vi "Write File.vi"(7 "File ID":string, 8 "error in (no error)":errorcluster, 9 "Segment 1 to 99":T3(array[cluster]), 10 "Segment 0":T2={"Start"=enum."Upward PV tart", "Cycle data"=999, "Pattern link data"=0, "Tag data"="PROG551A"}, 11 "Serial Config":T1={"串口选择"="", "通讯速率"=9600, "超时时间"=200, "数据位长"=8, "奇偶校验"=enum."None", "停止位长"=10, "握手控制"=0, "字符结束"=TRUE, "结束字符"=10, "仪器地址"=1} {"结束字符" format="%.0x"; "握手控制" items=["None", "XON/XOFF", "RTS/CTS", "XON/XOFF & RTS/CTS", "DTR/DSR", "XON/XOFF & DTR/DSR"]; "停止位长" items=["1.0"=10, "1.5"=15, "2.0"=20]; "数据位长" min=5 max=8 step=1}) -> (0 "error out":errorcluster)   [LabVIEW 2010, in "DCP551.lvlib"]
uses:
  DCP551.lvlib
  <vilib>/Instr/_visa.llb/VISA Configure Serial Port (Instr).vi
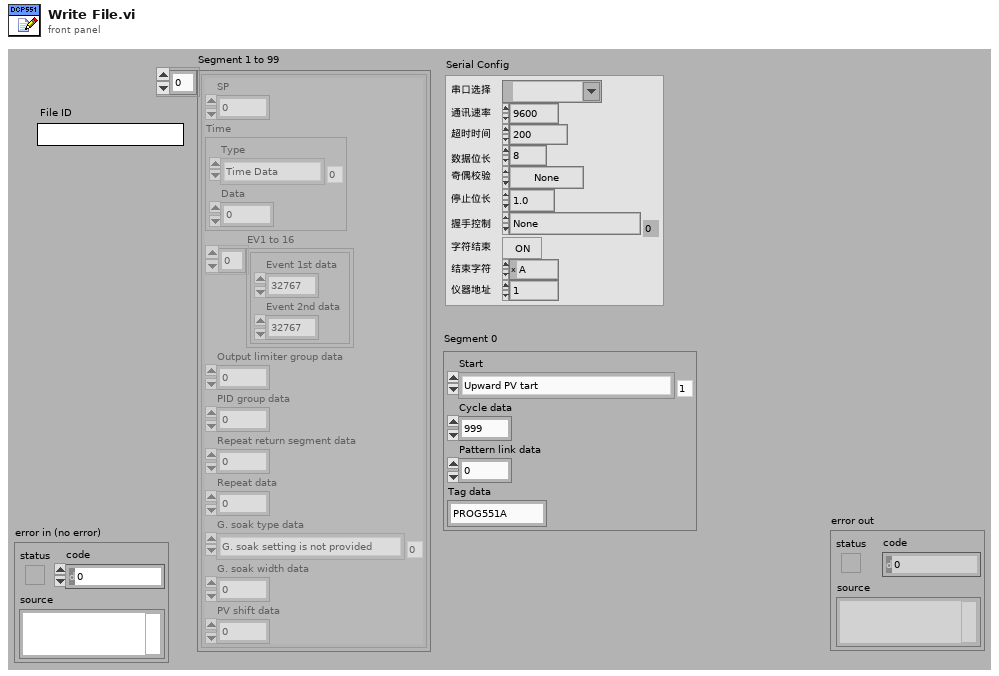
[diagram p1: front panel]
types:
  T1 = cluster{"串口选择":refnum<visa-resource-name>, "通讯速率":u32, "超时时间":u32, "数据位长":u16, "奇偶校验":enum16{"None", "Odd", "Even", "Mark", "Space"}, "停止位长":u16, "握手控制":u16, "字符结束":bool, "结束字符":u8, "仪器地址":u32}
  T2 = cluster{"Start":enum16{"Non PV start", "Upward PV tart", "Downward PV start", "Either upward of downward PV start"}, "Cycle data":i32, "Pattern link data":i32, "Tag data":string}
  T3 = cluster{"SP":dbl, "Time":cluster{"Type":enum16{"Time Data", "delta Dtada", "SP Data"}, "Data":i32}, "EV1 to 16":cluster{"Event 1st data":i32, "Event 2nd data":i32}[], "Output limiter group data":i32, "PID group data":i32, "Repeat return segment data":i32, "Repeat data":i32, "G. soak type data":enum16{"G. soak setting is not provided", "Segment start point", "Segment end point", "Total segment"}, "G. soak width data":i32, "PV shift data":i32}[]
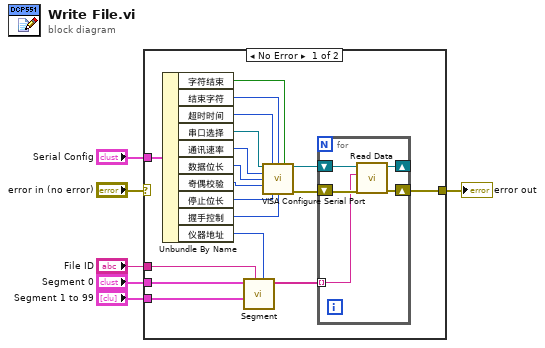
[diagram p0: block diagram]
diagram:
  n1 = case shown="No Error" "error in (no error)" {
    selector: "error in (no error)" -> [_ w30]
    tunnel: "Serial Config" -> [w15 _]
    tunnel: [w12 w30] -> w5
    tunnel: "Segment 1 to 99" -> [w10 _]
    tunnel: "Segment 0" -> [w11 _]
    tunnel: "File ID" -> [w9 _]
    frame No Error {
      n2 = Unbundle By Name(w15) -> ("字符结束"=w18:bool, "结束字符"=w17:u8, "超时时间"=w16:u32, "串口选择"=w24:refnum<visa-resource-name>, "通讯速率"=w23:u32, "数据位长"=w22:u16, "奇偶校验"=w21:enum16{"None", "Odd", "Even", "Mark", "Space"}, "停止位长"=w20:u16, "握手控制"=w19:u16, "仪器地址"=w8:u32)
      n3 = call "Segment.vi"("仪器地址"=w8, "File ID"=w9, "Segment 1 to 99"=w10, "Segment 0"=w11) -> ("Array"=w7:string[])  [unwired: 7 in]
      n4 = call-poly "VISA Configure Serial Port"("VISA resource name"=w24, "timeout (10sec)"=w16, "termination char\n(0xA = '\\n' = LF)"=w17, "Enable Termination\nChar (T)"=w18, "baud rate (9600)"=w23, "data bits (8)"=w22, "parity (0:none)"=w21, "stop bits (10: 1 bit)"=w20, "flow control (0:none)"=w19) -> ("VISA resource name out"=w14:refnum<visa-resource-name>, "error out"=w13:errorcluster)  [unwired: 1 in, 4 out]
      n5 = for {
        tunnel: w7 -> [w26] mode=indexing
        shift-right: [w27] -> w12
        shift-left: w13 -> [w28]
        shift-right: [w25] -> _
        shift-left: w14 -> [w29]
        n6 = call "Read Data.vi"("error in (no error)"=w28, "COMMAND"=w26, "VISA resource name in"=w29) -> ("error out"=w27:errorcluster, "VISA resource name out"=w25:refnum<visa-resource-name>)  [unwired: 6 in, 1 out]
      }
    }
    frame Error {
    }
  }
  "error out" <- w5
